vi "DC_Motor_Model.vi"() -> ()   [LabVIEW 2026]
panel:
  out "current":dbl(graph)=0.8
  in  "stop":bool
  in  "Time step":dbl=1e-05
  out "Torque":dbl(graph)=0.005272000000000001
  out "Speed":dbl(graph)=58.6284564098792
  out "Torque":dbl=0.005272000000000001
  out "Angular Speed":dbl=58.6284564098792
  out "Armature Current":dbl=0.8
  in  "Viscous Friction":dbl=0.00013
  in  "Rotor inertia":dbl=1e-07
  in  "Back EMF constant":dbl=0.006589
  in  "Torque Constant":dbl=0.00659
  in  "Armature inductance":dbl=7.5e-05
  in  "Armature resistance":dbl=3.41
  in  "Applied voltage":dbl=6.0
  # "the simulation dimonstrares the example of  brushed DC motor with permanent magnet with no load"
  # "Torque to current coeffitient for us is 1.46E+2"
  # "nearly matches datasheet"
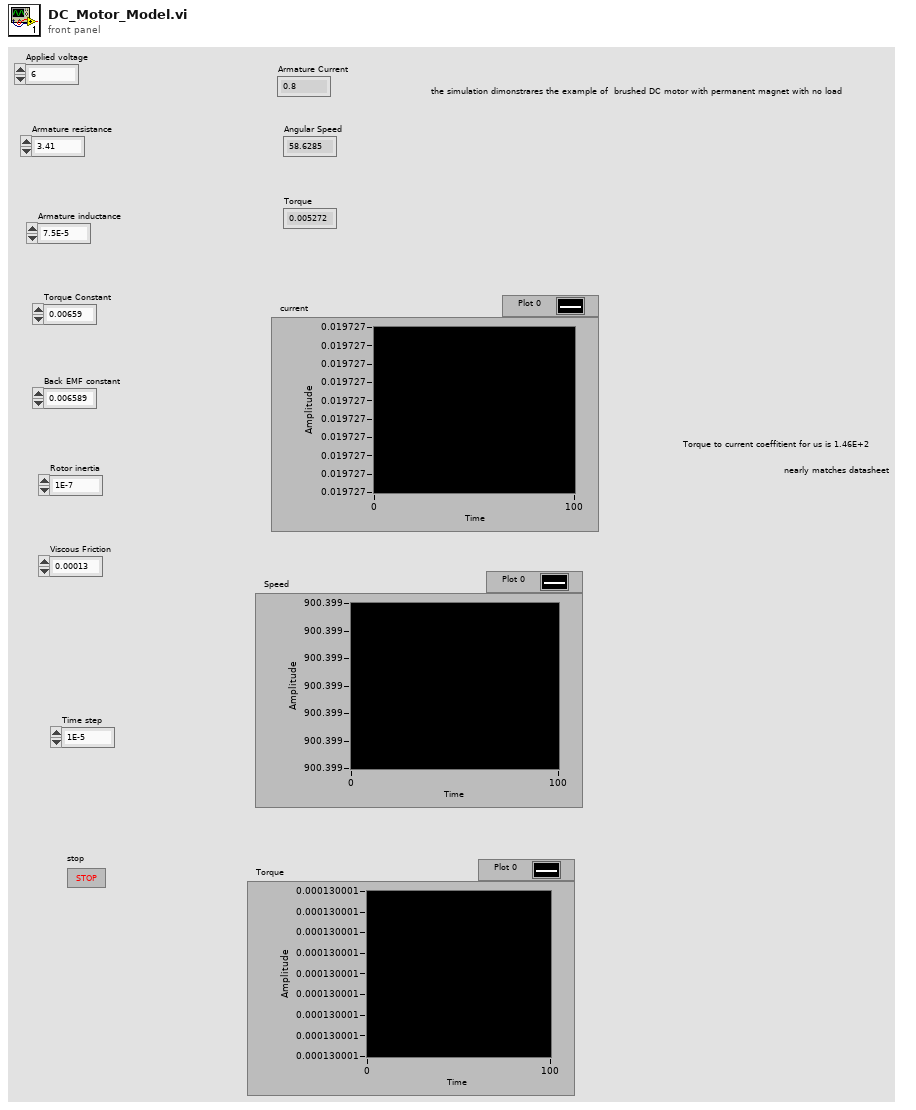
[diagram p1: front panel]
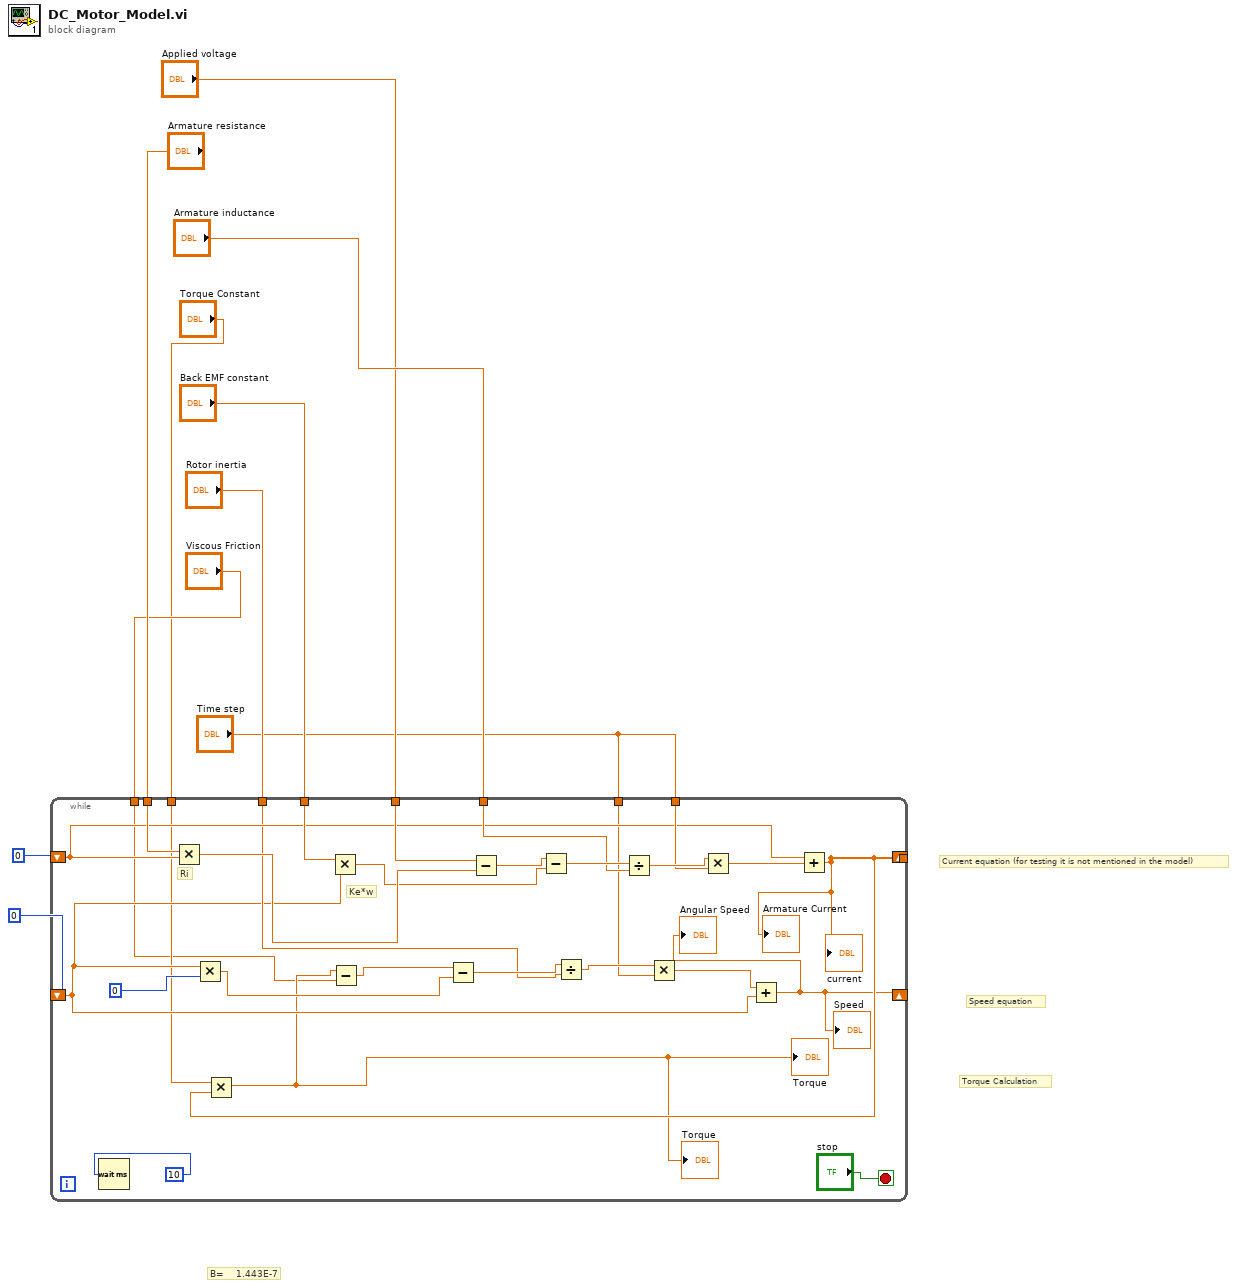
[diagram p0: block diagram]
diagram:
  # "B=    1.443E-7"
  # "Torque Calculation"
  # "Speed equation"
  # "Current equation (for testing it is not mentioned in the model)"
  n1 = while {
    shift-right: [w16] -> _
    shift-left: 0 -> [w28]
    shift-right: [w13] -> _
    shift-left: 0 -> [w18]
    tunnel: "Armature resistance" -> [w38]
    tunnel: "Back EMF constant" -> [w37]
    tunnel: "Applied voltage" -> [w36]
    tunnel: "Armature inductance" -> [w31]
    tunnel: "Time step" -> [w29]
    tunnel: [w16] -> _
    tunnel: "Viscous Friction" -> [w11]
    tunnel: "Rotor inertia" -> [w22]
    tunnel: "Time step" -> [w20]
    tunnel: "Torque Constant" -> [w17]
    stop <- "stop" stop-if-true
    # "Ke*w"
    # "Ri"
    n2 = Wait (ms)(milliseconds to wait=10 ("10")) -> ()  [unwired: 1 out]
    n3 = Multiply(x=w38, y=w28) -> (x*y=w35:dbl)
    n4 = Multiply(x=w18, y=0) -> (x*y=w15:dbl)
    n5 = Multiply(x=w37, y=w18) -> (x*y=w33:dbl)
    n6 = Subtract(x=w36, y=w35) -> (x-y=w34:dbl)
    n7 = Subtract(x=w34, y=w33) -> (x-y=w32:dbl)
    n8 = Divide(x=w32, y=w31) -> (x/y=w30:dbl)
    n9 = Multiply(x=w30, y=w29) -> (x*y=w27:dbl)
    n10 = Add(x=w28, y=w27) -> (x+y=w16:dbl)
    "Armature Current" <- w16
    "current" <- w16
    n11 = Multiply(x=w17, y=w16) -> (x*y=w12:dbl)
    "Torque" <- w12
    "Torque" <- w12
    n12 = Subtract(x=w12, y=w11) -> (x-y=w14:dbl)
    n13 = Subtract(x=w14, y=w15) -> (x-y=w23:dbl)
    n14 = Divide(x=w23, y=w22) -> (x/y=w21:dbl)
    n15 = Multiply(x=w21, y=w20) -> (x*y=w19:dbl)
    n16 = Add(x=w19, y=w18) -> (x+y=w13:dbl)
    "Speed" <- w13
    "Angular Speed" <- w13
  }
